vi "ErrorHandlingAfterShooting.vi"(6 "error in (no error)":errorcluster caption="entrée d'erreur (pas d'erreur)", 8 "Arduino Message IN":string, 9 "Nom de ressource VISA IN":refnum<visa-resource-name>) -> (0 "error out":errorcluster caption="sortie d'erreur", 1 "Arduino Message OUT":string, 2 "Try Shooting Again":bool, 3 "Nom de ressource VISA OUT":refnum<visa-resource-name>)   [LabVIEW 2014, in "ShootingStar.lvlib"]
uses:
  ShootingStar/ShootingStar.lvlib
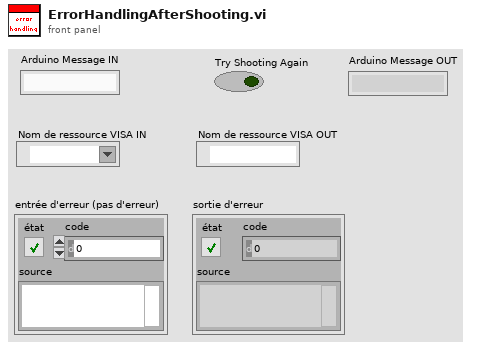
[diagram p1: front panel]
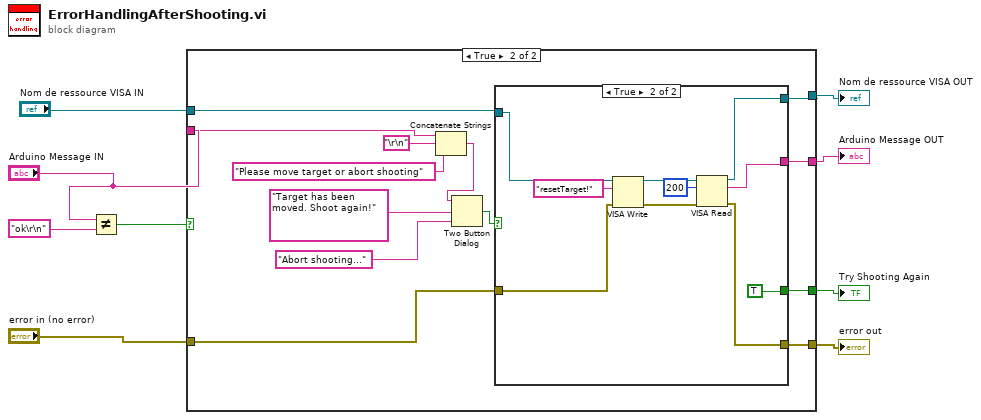
[diagram p0: block diagram]
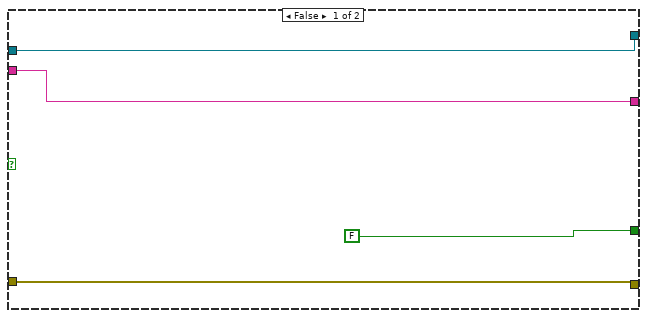
[diagram p2: hidden frame]
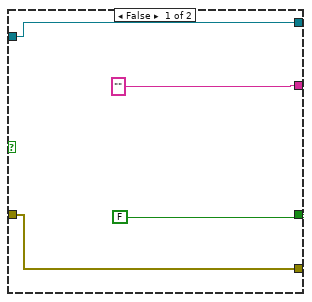
[diagram p3: hidden frame]
diagram:
  n1 = Not Equal?(x="Arduino Message IN", y="ok\r\n") -> (x != y?=w3:bool)
  n2 = case shown="True" w3 {
    tunnel: "Arduino Message IN" -> [w13 w26]
    tunnel: [w11 w19] -> w9
    tunnel: [w13 w18] -> w8
    tunnel: [w10 w17] -> w7
    tunnel: [FALSE w16] -> w6
    tunnel: "Nom de ressource VISA IN" -> [w10 w15]
    tunnel: "error in (no error)" -> [w11 w14]
    frame False {
    }
    frame True {
      n3 = Concatenate Strings(w26, "\r\n", "Please move target or abort shooting" ("message")) -> (w21:string)
      n4 = Two Button Dialog(message=w21, 1:"Abort shooting..." ("Nom du bouton F (\"Annuler\")"), 2:"Target has been moved. Shoot again!" ("Nom du bouton V (\"OK\")")) -> (T button?=w20:bool)
      n5 = case shown="True" w20 {
        tunnel: w15 -> [w30 w40]
        tunnel: w14 -> [w28 w38]
        tunnel: [w28 w34] -> w19
        tunnel: ["" ("read buffer") w33] -> w18
        tunnel: [w30 w32] -> w17
        tunnel: [FALSE TRUE] -> w16
        frame False {
        }
        frame True {
          n6 = VISA Write(VISA resource name=w40, write buffer="resetTarget!" ("buffer d'écriture"), error in (no error)=w38) -> (VISA resource name out=w37:refnum<visa-resource-name>, error out=w35:errorcluster)  [unwired: 1 out]
          n7 = VISA Read(VISA resource name=w37, byte count=u32 200 ("nombre d'octets"), error in (no error)=w35) -> (VISA resource name out=w32:refnum<visa-resource-name>, read buffer=w33:string, error out=w34:errorcluster)  [unwired: 1 out]
        }
      }
    }
  }
  "Try Shooting Again" <- w6
  "Nom de ressource VISA OUT" <- w7
  "error out" <- w9
  "Arduino Message OUT" <- w8
